vi "Python_TransferFile.vi"(8 "File text":string, 9 "File name":string, 10 "Python version":string="3.9", 11 "Port":string) -> (2 "Console":string)   [LabVIEW 2020]
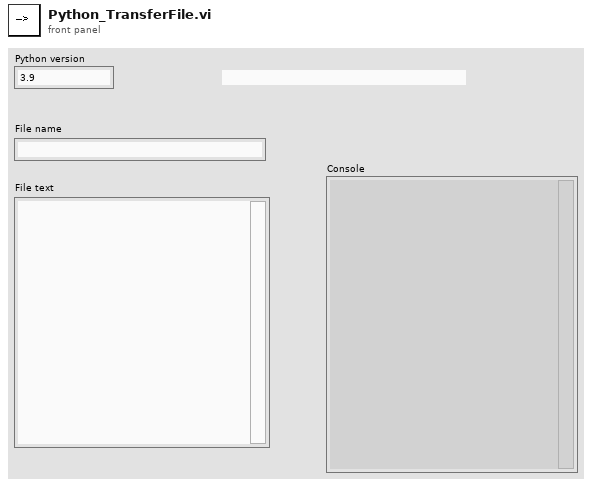
[diagram p1: front panel]
types:
  T1 = typedef "PythonCtrl.ctl" = cluster{"session":refnum<k35>, "PyPath":path}
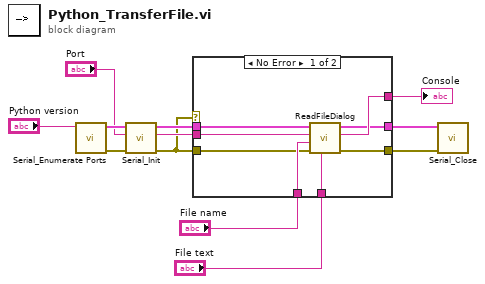
[diagram p0: block diagram]
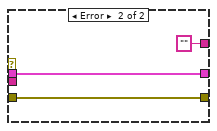
[diagram p2: hidden frame]
diagram:
  n1 = call "Serial_Enumerate Ports.vi"("Python version"="Python version") -> ("error out"=w10:errorcluster, "Python"=w12:T1)  [unwired: 7 in, 2 out]
  n2 = call "Serial_Init.vi"("error in (no error)"=w10, "Port"="Port", "Python"=w12) -> ("error out"=w2:errorcluster, "Console"=w7:string, "Python out"=w8:T1)  [unwired: 6 in]
  n3 = case shown="No Error" w2 {
    tunnel: w8 -> [w16 w22]
    tunnel: w2 -> [w14 w21]
    tunnel: w7 -> [w15 _]
    tunnel: "File name" -> [w19 _]
    tunnel: [w18 w21] -> w5
    tunnel: [w16 w22] -> w4
    tunnel: [w17 "" ("Console")] -> w3
    tunnel: "File text" -> [w13 _]
    frame No Error {
      n4 = call "ReadFileDialog.vi"("File Text"=w13, "error in (no error)"=w14, "File name"=w19, "Console in"=w15, "Python in"=w16) -> ("error out"=w18:errorcluster, "Console"=w17:string)  [unwired: 5 in]
    }
    frame Error {
    }
  }
  "Console" <- w3
  n5 = call "Serial_Close.vi"("error in (no error)"=w5, "Python in"=w4) -> ()  [unwired: 10 in]
